vi "FdxCmdMonQueueRead(native).vi"(6 "MaxReadBytes":u32=65535, 8 "error in":errorcluster, 9 "EntryCount":u32=1, 10 "QueueId":u32, 11 "InstrumentHandle_port":u32) -> (0 "error out":errorcluster, 1 "QueueReadOut":T1, 2 "QueueIdOut":u32, 3 "InstrumentHandle_port":u32)   [LabVIEW 2020]
doc: "This function is used to read Entries of a chronological capturing queue to a provided buffer. For this read function only the number of Entries to be read is specified. The reading start position is administrated internal to the target. The start position can by identified and modified by the functions AiFdxCmdMonQueueTell(...) and AiFdxCmdMonQueueSeek(...). Additional processing, for accessing the Frame Header data must be done via AiFdxProcessMonQueue function.\nNote: Data, read via AiFdxCmdMonQueueRead, can be directly used for Replay via the AiFdxCmdTxQueueWrite function, if the corresponding Transmit Port has been configured for Replay."
uses:
  <instrlib>/AIM GmbH/_AIM 664/bsp/LIbraryAdmin/FdxGlobalDllPath.vi
  <instrlib>/AIM GmbH/_AIM 664/bsp/LIbraryAdmin/FdxGetErrorDescription.vi
  <vilib>/Utility/error.llb/Error Cluster From Error Code.vi
  <instrlib>/AIM GmbH/_AIM 664/AIM664LV.lvlib
panel:
  in  "ReadQualifier":u32(ring) items=["FDX_MON_READ_FULL", "FDX_MON_READ_HEADER", "FDX_MON_READ_DATA"]
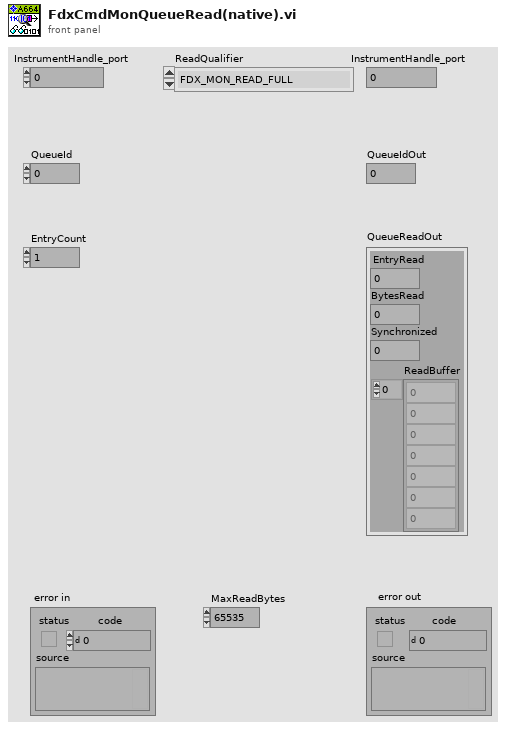
[diagram p1: front panel]
types:
  T1 = cluster{"EntryRead":u32, "BytesRead":u32, "Synchronized":u32, "ReadBuffer":u8[]}
  T2 = cluster{"ul_EntryRead":u32, "ul_BytesRead":u32, "ul_Synchronized":u32, "vpv_ReadBuffer":u64}
  T3 = cluster{"ul_EntryCount":u32, "ul_ReadQualifier":u32, "ul_MaxReadBytes":u32}
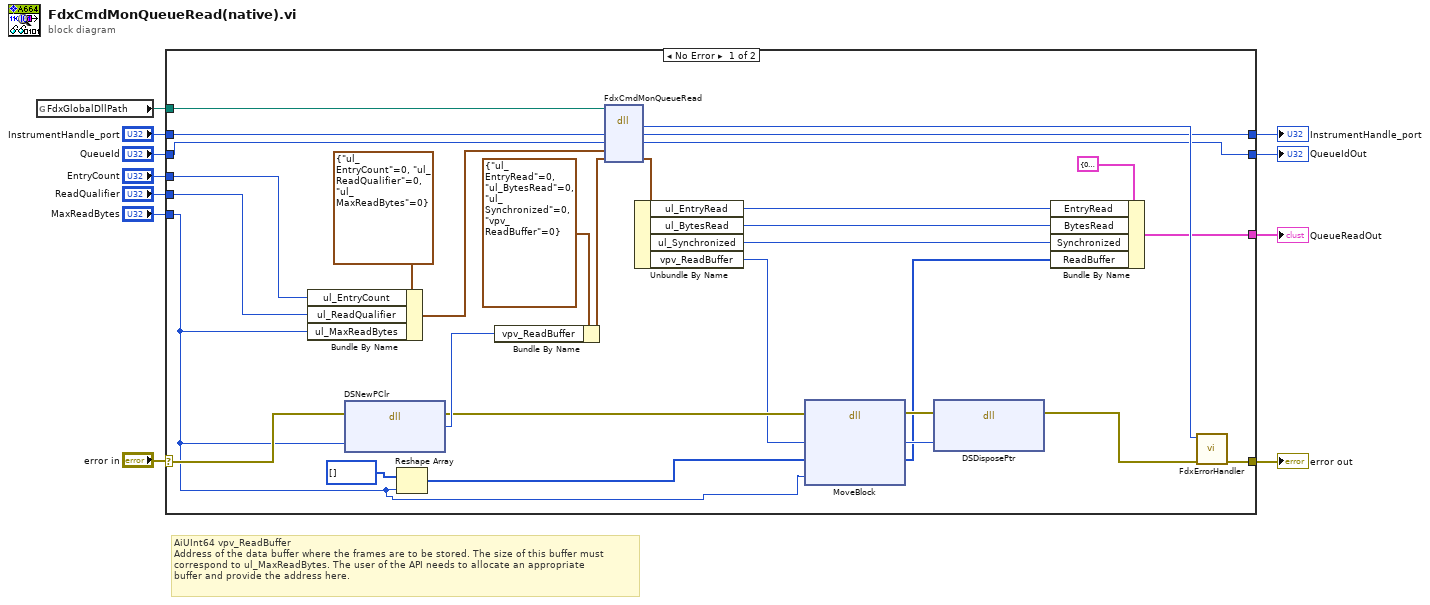
[diagram p0: block diagram]
diagram:
  # "AiUInt64 vpv_ReadBuffer\nAddress of the data buffer where the frames are to be stored. The size of this buffer must\ncorrespond to ul_MaxReadBytes. The user of the API needs to allocate an appropriate\nbuffer and provide the address here."
  n1 = global read "FdxGlobalDllPath.vi" "FdxGlobalDllPath"() -> (w9:path)
  n2 = case shown="No Error" "error in" {
    selector: "error in" -> [w22 w44]
    tunnel: [w41 w44] -> w11
    tunnel: w9 -> [w39 _]
    tunnel: "InstrumentHandle_port" -> [w38 w43]
    tunnel: [w37 w43] -> w7
    tunnel: "QueueId" -> [w36 w42]
    tunnel: "EntryCount" -> [w33 _]
    tunnel: "ReadQualifier" -> [w32 _]
    tunnel: "MaxReadBytes" -> [w14 _]
    tunnel: [w35 w42] -> w2
    tunnel: [w28 _] -> w1
    frame No Error {
      n3 = Bundle By Name(cluster=T3 {"ul_EntryCount"=0, "ul_ReadQualifier"=0, "ul_MaxReadBytes"=0}, "ul_EntryCount"=w33, "ul_ReadQualifier"=w32, "ul_MaxReadBytes"=w14) -> (w31:T3)
      n4 = dll-call lib="LabVIEW" fn="DSNewPClr"(error in=w22, "size"=w14) -> (error out=w18:errorcluster, "pointer"=w21:u64)  [unwired: 3 in, 1 out]
      n5 = Reshape Array(u8[] [] ("buffer in"), w14) -> (w15:u8[])
      n6 = Bundle By Name(cluster=T2 {"ul_EntryRead"=0, "ul_BytesRead"=0, "ul_Synchronized"=0, "vpv_ReadBuffer"=0}, "vpv_ReadBuffer"=w21) -> (w23:T2)
      n7 = dll-call lib="aim_fdx.19.dll" fn="FdxCmdMonQueueRead"(path in=w39, "ul_Handle"=w38, "ul_QueueId"=w36, "px_QueueReadIn"=w31, "px_QueueReadOut"=w23) -> ("status"=w40:i32, "ul_Handle"=w37:u32, "ul_QueueId"=w35:u32, "px_QueueReadOut"=w27:T2)  [unwired: 3 in, 2 out]
      n8 = Unbundle By Name(w27) -> ("ul_EntryRead"=w26:u32, "ul_BytesRead"=w25:u32, "ul_Synchronized"=w24:u32, "vpv_ReadBuffer"=w16:u64)
      n9 = dll-call lib="LabVIEW" fn="MoveBlock"(error in=w18, "src"=w16, "dst"=w15, "size"=w14) -> (error out=w17:errorcluster, "src"=w13:u64, "dst"=w12:u8[])  [unwired: 4 in, 1 out]
      n10 = dll-call lib="LabVIEW" fn="DSDisposePtr"(error in=w17, "pointer"=w13) -> (error out=w20:errorcluster)  [unwired: 4 in, 1 out]
      n11 = Bundle By Name(cluster=T1 {"EntryRead"=0, "BytesRead"=0, "Synchronized"=0, "ReadBuffer"=[]} ("QueueReadOut"), "EntryRead"=w26, "BytesRead"=w25, "Synchronized"=w24, "ReadBuffer"=w12) -> (w28:T1)
      n12 = call <instrlib>:"FdxErrorHandler.vi"("error in"=w20, "AIM Error"=w40) -> ("error out"=w41:errorcluster)  [unwired: 9 in]
    }
    frame Error {
    }
  }
  "error out" <- w11
  "InstrumentHandle_port" <- w7
  "QueueIdOut" <- w2
  "QueueReadOut" <- w1
